vi "PropertyAdd.vi"(0 "Data":T1, 5 "error in":errorcluster) -> (14 "Data 2":T1, 19 "error out":errorcluster)   [LabVIEW 2017]
doc: "<B>This VI is used for adding a new property to the Caps file.</B>"
uses:
  Ctrl/Type Tab.ctl
  Ctrl/compond commands.ctl
  Ctrl/User Input Cluster.ctl
  Ctrl/Property.ctl
  Ctrl/PhysicalChannel.ctl
  Ctrl/Bitfield.ctl
  Ctrl/Register.ctl
  Ctrl/ScaleType.ctl
  Ctrl/Scale.ctl
  Ctrl/EnumValue.ctl
  Ctrl/Enum.ctl
  Ctrl/Caps.ctl
  Ctrl/Data.ctl
panel:
  in  "Write a Range?":bool
  out "Lable":string
  in  "Write a Register?":bool
  in  "Scale method":u16(ring) items=["TableStrict", "TableStrict12Elements", "PolynomialBoundaryConditions", "PolynomialThermocouple", "Times2Plus2", "LinearDivideBy8", "TableInterpolate", "TableRound", "NoScale"]
  in  "Min":dbl
  in  "Max":dbl
  out "Data Range":T11
  in  "Min(Double)":dbl
  in  "Max(Double)":dbl
  in  "Max(U64)":u64
  in  "Min(U64)":u64
  in  "Min(I64)":i64
  in  "Max(I64)":i64
  in  "Max(U32)":u32
  in  "Min(U32)":u32
  in  "Min(I32)":i32
  in  "Max(I32)":i32
  in  "OK Button":bool
  in  "Documentation":string
  in  "String":string
  in  "U8":u8 format="%.0x"
  in  "I8":i8
  in  "U32":u32
  in  "I32":i32
  in  "U64":u64
  in  "I64":i64
  in  "Ring":u16(ring) items=["False", "True"]
  in  "DBL":dbl format="%#_16g"
  in  "Description":string
  in  "Access":u16(ring) items=["Read Only", "Write Only", "Read/Write"]
  in  "Bitfield":u16(ring) items=["DebugScratch8/ScratchI8", "DebugScratch8/Scratch8", "DebugScratch8/ScratchBool", "DebugScratch16/ScratchBool", "DebugScratch16/ScratchI8", "DebugScratch16/Scratch8", "DebugScratch16/ScratchI16", "DebugScratch16/Scratch16", "DebugScratch32/ScratchBool", "DebugScratch32/ScratchI8", "DebugScratch32/Scratch8", "DebugScratch32/ScratchI16", "DebugScratch32/Scratch16", "DebugScratch32/ScratchI32", "DebugScratch32/Scratch32", "DebugLeds/DebugLed3", "DebugLeds/DebugLed2", "DebugLeds/DebugLed1", "DebugLeds/DebugLed0", "DebugDipSwitch/DipSwitch8", "DebugDipSwitch/DipSwitch7", "DebugDipSwitch/DipSwitch6", "DebugDipSwitch/DipSwitch5", "DebugDipSwitch/DipSwitch4", "DebugDipSwitch/DipSwitch3", "DebugDipSwitch/DipSwitch2", "DebugDipSwitch/DipSwitch1", "DebugScratch64/ScratchBool", "DebugScratch64/ScratchI8", "DebugScratch64/Scratch8", "DebugScratch64/ScratchI16", "DebugScratch64/Scratch16", "DebugScratch64/ScratchI32", "DebugScratch64/Scratch32", "DebugScratch64/ScratchI64", "DebugScratch64/Scratch64", "FrontPanelLeds/LedRed0Enable", "FrontPanelLeds/LedRed1Enable", "FrontPanelLeds/LedRed2Enable", "FrontPanelLeds/LedGreen0Enable", "FrontPanelLeds/LedGreen1Enable", "FrontPanelLeds/LedGreen2Enable", "Revision/DateCode", "InterruptAck/EventIntAck0", "InterruptAck/EventIntAck1", "InterruptAck/EventIntAck2", "InterruptAck/EventIntAck3", "InterruptAck/ExternalIntAck0", "InterruptAck/ExternalIntAck1", "InterruptAck/ExternalIntAck2", "InterruptAck/ExternalIntAck3", "InterruptDisable/EventIntDisable0", "InterruptDisable/EventIntDisable1", "InterruptDisable/EventIntDisable2", "InterruptDisable/EventIntDisable3", "InterruptDisable/ExternalIntDisable0", "InterruptDisable/ExternalIntDisable1", "InterruptDisable/ExternalIntDisable2", "InterruptDisable/ExternalIntDisable3", "InterruptEnable/EventIntEnable0", "InterruptEnable/EventIntEnable1", "InterruptEnable/EventIntEnable2", "InterruptEnable/EventIntEnable3", "InterruptEnable/ExternalIntEnable0", "InterruptEnable/ExternalIntEnable1", "InterruptEnable/ExternalIntEnable2", "InterruptEnable/ExternalIntEnable3", "InterruptMask/EventIntMask0", "InterruptMask/EventIntMask1", "InterruptMask/EventIntMask2", "InterruptMask/EventIntMask3", "InterruptMask/ExternalIntMask0", "InterruptMask/ExternalIntMask1", "InterruptMask/ExternalIntMask2", "InterruptMask/ExternalIntMask3", "InterruptStatus/EventIntStatus0", "InterruptStatus/EventIntStatus1", "InterruptStatus/EventIntStatus2", "InterruptStatus/EventIntStatus3", "InterruptStatus/ExternalIntStatus0", "InterruptStatus/ExternalIntStatus1", "InterruptStatus/ExternalIntStatus2", "InterruptStatus/ExternalIntStatus3", "EventCounter3/DelayInMilliseconds", "EventCounter2/DelayInMilliseconds", "EventCounter1/DelayInMilliseconds", "EventCounter0/DelayInMilliseconds", "EventStartRegister/EventStart0", "EventStartRegister/EventStart1", "EventStartRegister/EventStart2", "EventStartRegister/EventStart3"]
  in  "DataType":T12(ring)
  in  "Name":string
  # "Value"
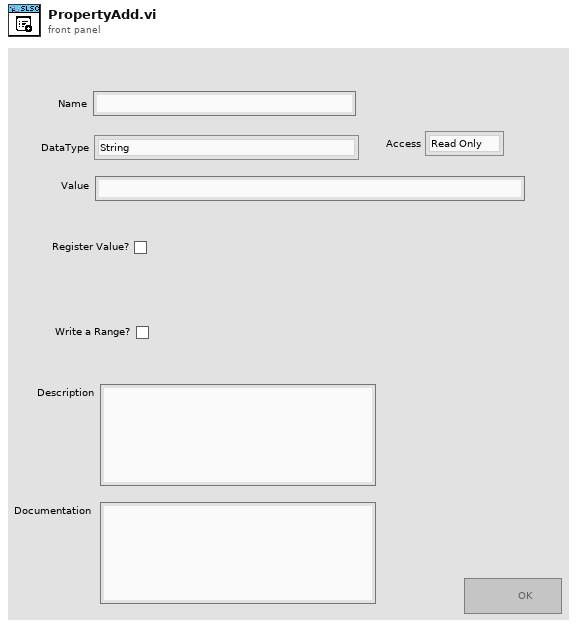
[diagram p1: front panel]
types:
  T1 = typedef "Data.ctl" = cluster{"Ref Cluster":cluster{"String":refnum<vi>, "U8":refnum<vi>, "I8":refnum<vi>, "U32":refnum<vi>, "I32":refnum<vi>, "U64":refnum<vi>, "I64":refnum<vi>, "Ring":refnum<vi>, "DBL":refnum<vi>, "Add":refnum<vi>, "Remove":refnum<vi>, "Property tree":refnum<vi>}, "JSON Text":string, "Original JSON Text":string, "Caps":T2, "SLSC Output Tree":cluster{"Left Cell String":string, "Child Text":string[], "Child Tag":string, "Item Indent":i32, "Child Only?":bool, "Glyph Index":i32, "offline value":variant}[], "Ref Index and Control Type":cluster{"index":i32, "Datatype":string}, "Selected Type and name":cluster{"Selected Type":enum16{"Property", "Physical Channel"}, "Selected Property Name":string}, "Update whole Tree?":bool}
  T2 = typedef "Caps.ctl" = cluster{"properties":T3[], "physical channels":T4[], "registers":T5[], "scales":T7[], "enums":T9[], "productName":string}
  T3 = typedef "Property.ctl" = cluster{"name":string, "bitfield":string, "value":variant, "dataType":string, "min":variant, "max":variant, "scale":string, "access":string}
  T4 = typedef "PhysicalChannel.ctl" = cluster{"name":string, "properties":T3[]}
  T5 = typedef "Register.ctl" = cluster{"name":string, "address":i32, "size":i32, "bitfields":T6[], "initialValue":variant, "connectedProperties":string[]}
  T6 = typedef "Bitfield.ctl" = cluster{"name":string, "offset":i32, "size":i32, "signed":bool}
  T7 = typedef "Scale.ctl" = cluster{"name":string, "type":T8, "params":variant}
  T8 = typedef "ScaleType.ctl" = enum16{"NoScale", "Table", "Polynomial", "Linear"}
  T9 = typedef "Enum.ctl" = cluster{"name":string, "values":T10[]}
  T10 = typedef "EnumValue.ctl" = cluster{"name":string, "value":i32}
  T11 = typedef "Type Tab.ctl" = enum32{"String", "Double", "U64", "I64", "U32", "I32", "Bool"}
  T12 = enum16{"String", "Double", "U64", "I64", "U32", "I32", "Bool"}
  T13 = typedef "User Input Cluster.ctl" = cluster{"Name":string, "DataType":enum16{"String", "Double", "U64", "I64", "U32", "I32", "Bool"}, "Bitfield":u16, "Access":u16, "Description":string, "Documentation":string, "Min_Max_Cluster":cluster{"Min(Double)":dbl, "Max(Double)":dbl, "Min(U64)":u64, "Max(U64)":u64, "Min(I64)":i64, "Max(I64)":i64, "Min(U32)":u32, "Max(U32)":u32, "Min(I32)":i32, "Max(I32)":i32}, "Value Cluster":cluster{"DBL":dbl, "Ring":u16, "I64":i64, "U64":u64, "I32":i32, "U32":u32, "I8":i8, "U8":u8, "String":string}, "Scale method list":u16}
  T14 = cluster{"DBL":dbl, "Ring":u16, "I64":i64, "U64":u64, "I32":i32, "U32":u32, "I8":i8, "U8":u8, "String":string}
  T15 = cluster{"Min(Double)":dbl, "Max(Double)":dbl, "Min(U64)":u64, "Max(U64)":u64, "Min(I64)":i64, "Max(I64)":i64, "Min(U32)":u32, "Max(U32)":u32, "Min(I32)":i32, "Max(I32)":i32}
  T16 = enum8{"Enabled", "Disabled", "Disabled and Grayed Out"}
  T17 = typedef "compond commands.ctl" = enum16{"Get Property Array", "Get Physical Channel Property Array", "Get the Selected Position", "Get Property and Physical Channel Name", "Get Type and Value", "Make and Set a new Property", "Modify the Value", "Delete a Property"}
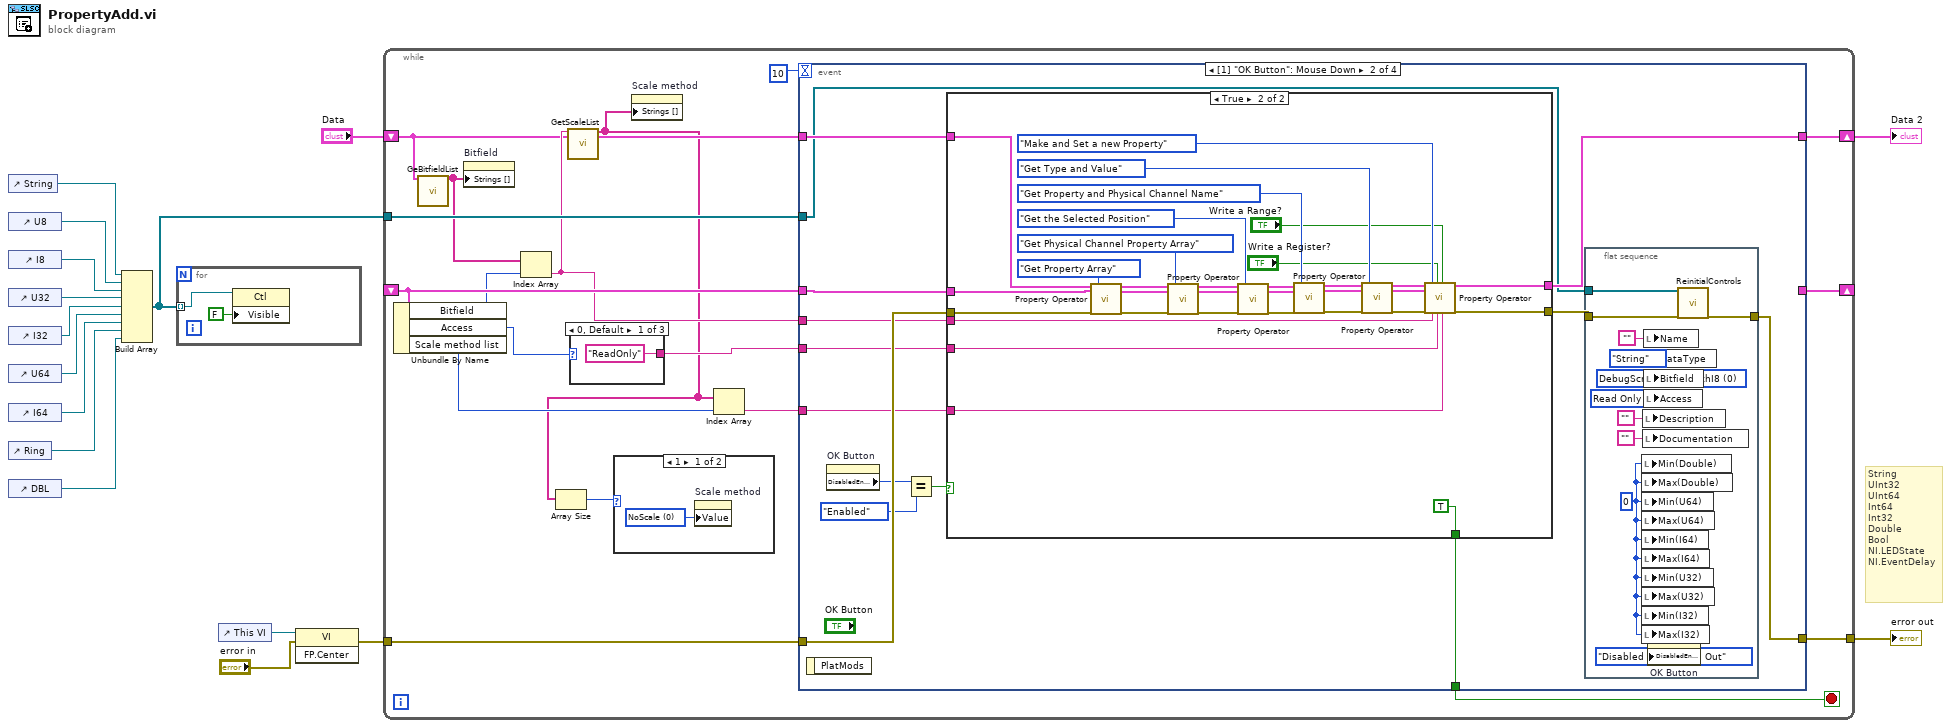
[diagram p0: block diagram]
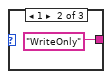
[diagram p3: hidden frame]
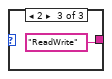
[diagram p4: hidden frame]
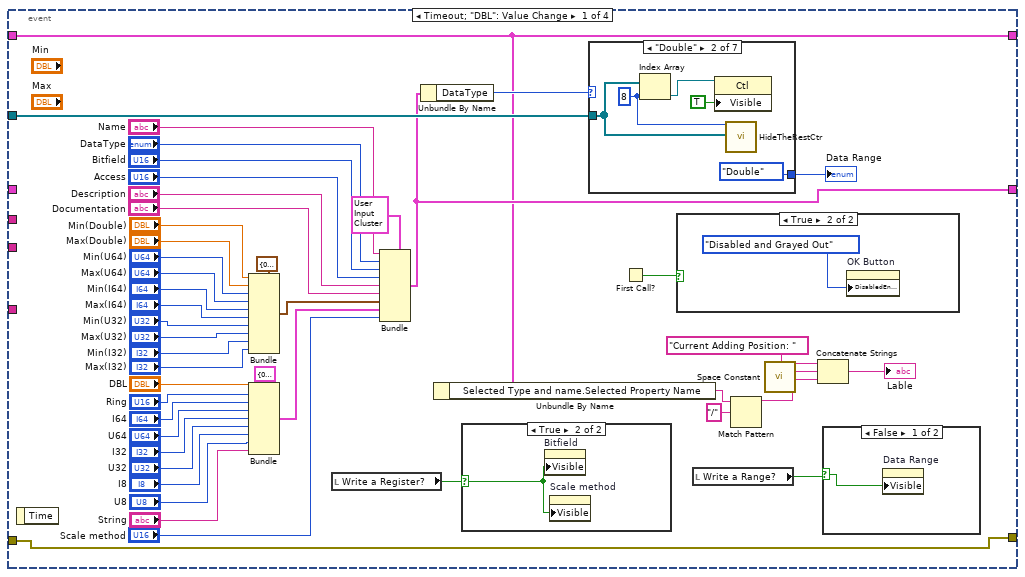
[diagram p5: hidden frame]
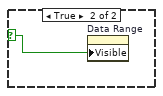
[diagram p6: hidden frame]
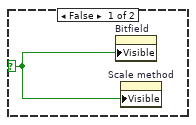
[diagram p7: hidden frame]
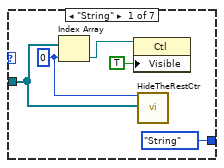
[diagram p9: hidden frame]
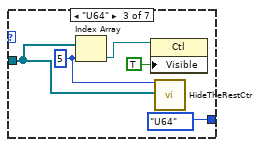
[diagram p10: hidden frame]
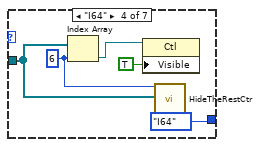
[diagram p11: hidden frame]
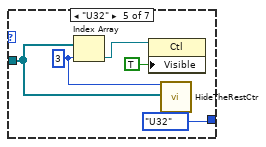
[diagram p12: hidden frame]
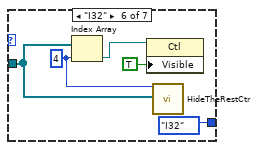
[diagram p13: hidden frame]
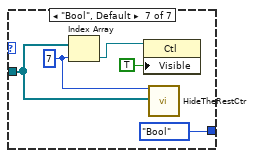
[diagram p14: hidden frame]
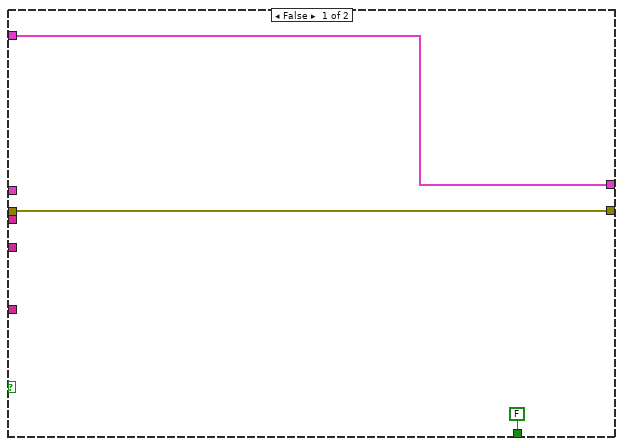
[diagram p15: hidden frame]
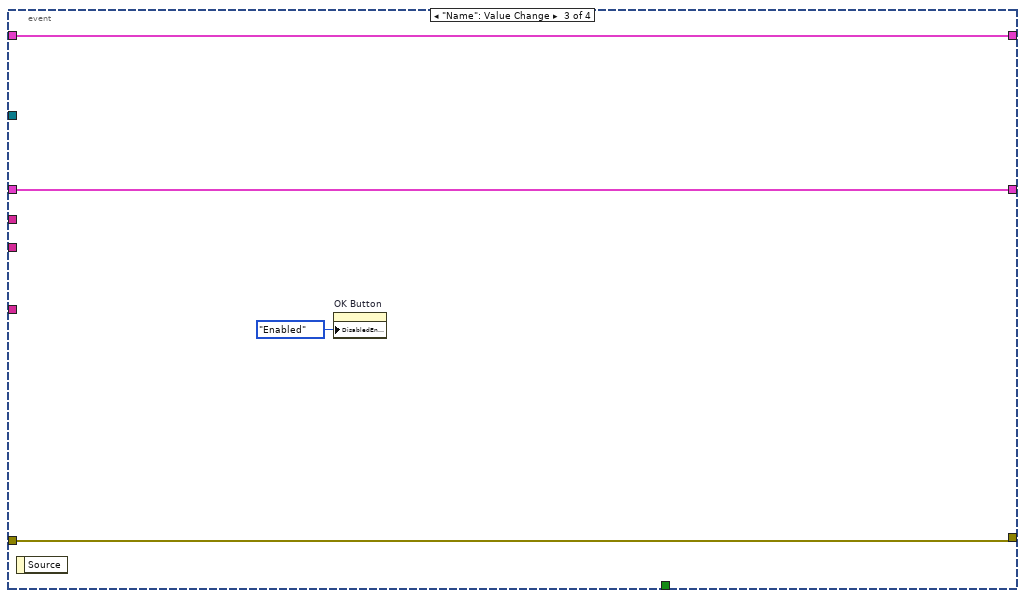
[diagram p16: hidden frame]
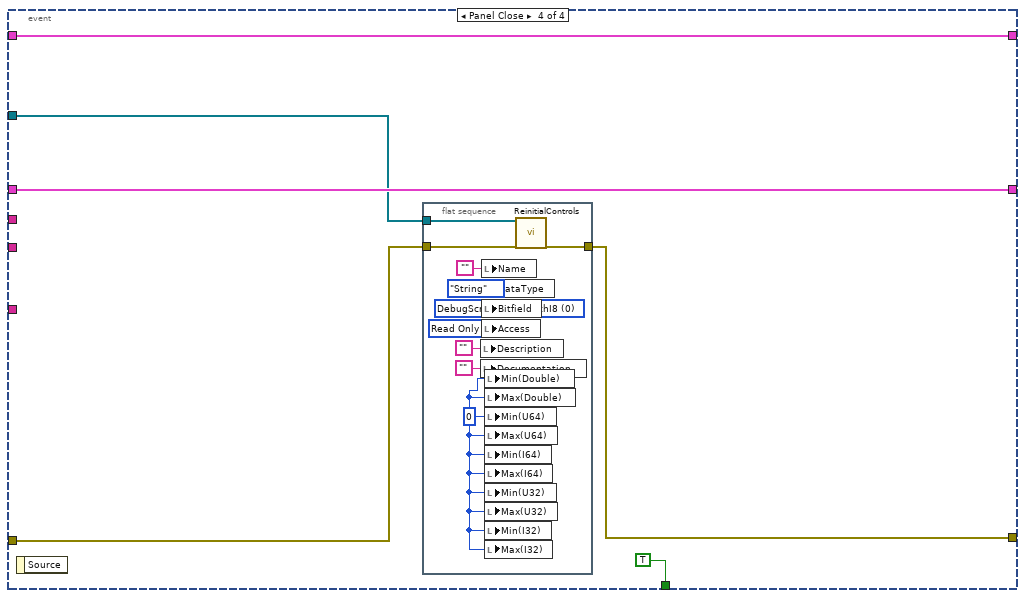
[diagram p17: hidden frame]
diagram:
  # "String\nUInt32\nUInt64\nInt64\nInt32\nDouble\nBool\nNI.LEDState\nNI.EventDelay"
  n1 = control-ref of="String"() -> (w16:refnum<vi>)
  n2 = control-ref of="U8"() -> (w15:refnum<vi>)
  n3 = control-ref of="I8"() -> (w14:refnum<vi>)
  n4 = control-ref of="U32"() -> (w13:refnum<vi>)
  n5 = control-ref of="I32"() -> (w12:refnum<vi>)
  n6 = control-ref of="U64"() -> (w11:refnum<vi>)
  n7 = control-ref of="I64"() -> (w10:refnum<vi>)
  n8 = control-ref of="Ring"() -> (w9:refnum<vi>)
  n9 = control-ref of="DBL"() -> (w8:refnum<vi>)
  n10 = Build Array(w16, w15, w14, w13, w12, w11, w10, w9, w8) -> (w1:refnum<vi>[])
  n11 = for {
    tunnel: w1 -> [w18] mode=indexing
    n12 = property class="Ctl"(reference=w18, "Visible"=FALSE) -> ()  [unwired: 1 in, 2 out]
  }
  n13 = control-ref of="This VI"() -> (w4:refnum<vi>)
  n14 = invoke class="VI" method="FP.Center"(reference=w4, error in="error in") -> (error out=w3:errorcluster)  [unwired: 1 in, 2 out]
  n15 = while {
    tunnel: w1 -> [w34]
    tunnel: w3 -> [w35]
    tunnel: [w36] -> w7
    shift-right: [w37] -> w5
    shift-left: "Data" -> [w25]
    shift-right: [w32] -> _
    shift-left: _ -> [w31]
    stop <- w19 stop-if-true
    n16 = Unbundle By Name(w31) -> ("Bitfield"=w30:u16, "Access"=w29:u16, "Scale method list"=w23:u16)
    n17 = call "GeBitfieldList.vi"("Data"=w25) -> ("Array"=w24:string[])  [unwired: 18 in]
    n18 = property on="Bitfield" class="Ring (strict)"("Strings []"=w24) -> ()  [unwired: 2 in, 2 out]
    n19 = Index Array(array=w24, index=w30) -> (element=w28:string)
    n20 = call "GetScaleList.vi"("Bitfield in"=w28, "Data in"=w25) -> ("output array"=w21:string[], "Data out"=w26:T1)  [unwired: 16 in]
    n21 = Array Size(array=w21) -> (size(s)=w20:i32)
    n22 = case shown="0, Default" w29 {
      tunnel: ["ReadOnly" "WriteOnly" "ReadWrite"] -> w27
      frame 0, Default {
      }
      frame 1 {
      }
      frame 2 {
      }
    }
    n23 = case shown="1" w20 {
      frame 1 {
        w38 = u16 0 items=["NoScale"] ("Scale method")
        n24 = property on="Scale method" class="Ring (strict)"("Value"=w38) -> ()  [unwired: 2 in, 2 out]
      }
      frame Default {
      }
    }
    n25 = property on="Scale method" class="Ring (strict)"("Strings []"=w21) -> ()  [unwired: 2 in, 2 out]
    n26 = Index Array(array=w21, index=w23) -> (element=w22:string)
    n27 = event shown="[1] \"OK Button\": Mouse Down" {
      selector: _ -> [_ _ _ _]
      dyn-events: _ -> [_ _ _ _]
      timeout: 10 -> [_ _ _ _]
      tunnel: w26 -> [w50 w140 w191 w197]
      tunnel: [w50 w139 w191 w197] -> w37
      tunnel: w35 -> [w51 w141 w188 w194]
      tunnel: [w51 w137 w188 w193] -> w36
      tunnel: w31 -> [_ w135 w190 w196]
      tunnel: w34 -> [w85 w136 _ w195]
      tunnel: [w56 _ w190 w196] -> w32
      tunnel: w28 -> [_ w134 _ _]
      tunnel: w27 -> [_ w133 _ _]
      tunnel: w22 -> [_ w132 _ _]
      tunnel: [_ w128 _ TRUE] -> w19
      event Timeout; "DBL": Value Change {
        n28 = event-data() -> ()  [unwired: 1 in, 1 out]
        n29 = Bundle(cluster=T15 {"Min(Double)"=0.0, "Max(Double)"=0.0, "Min(U64)"=0, "Max(U64)"=0, "Min(I64)"=0, "Max(I64)"=0, "Min(U32)"=0, "Max(U32)"=0, "Min(I32)"=0, "Max(I32)"=0} ("Min_Max_Cluster"), "Min(Double)"="Min(Double)", "Max(Double)"="Max(Double)", "Min(U64)"="Min(U64)", "Max(U64)"="Max(U64)", "Min(I64)"="Min(I64)", "Max(I64)"="Max(I64)", "Min(U32)"="Min(U32)", "Max(U32)"="Max(U32)", "Min(I32)"="Min(I32)", "Max(I32)"="Max(I32)") -> (w60:T15)
        n30 = Bundle(cluster=T14 {"DBL"=0.0, "Ring"=0, "I64"=0, "U64"=0, "I32"=0, "U32"=0, "I8"=0, "U8"=0, "String"=""} ("Value Cluster"), "DBL"="DBL", "Ring"="Ring", "I64"="I64", "U64"="U64", "I32"="I32", "U32"="U32", "I8"="I8", "U8"="U8", "String"="String") -> (w59:T14)
        n31 = local read "Write a Register?"() -> (w49:bool)
        n32 = Bundle(cluster=T13 {"Name"="", "DataType"=enum."String", "Bitfield"=0, "Access"=0, "Description"="", "Documentation"="", "Min_Max_Cluster"={"Min(Double)"=0.0, "Max(Double)"=0.0, "Min(U64)"=0, "Max(U64)"=0, "Min(I64)"=0, "Max(I64)"=0, "Min(U32)"=0, "Max(U32)"=0, "Min(I32)"=0, "Max(I32)"=0}, "Value Cluster"={"DBL"=0.0, "Ring"=0, "I64"=0, "U64"=0, "I32"=0, "U32"=0, "I8"=0, "U8"=0, "String"=""}, "Scale method list"=0}, "Name"="Name", "DataType"="DataType", "Bitfield"="Bitfield", "Access"="Access", "Description"="Description", "Documentation"="Documentation", "Min_Max_Cluster"=w60, "Value Cluster"=w59, "Scale method list"="Scale method") -> (w56:T13)
        n33 = Unbundle By Name(w56) -> ("DataType"=w86:T12)
        n34 = Unbundle By Name(w50) -> ("Selected Type and name.Selected Property Name"=w45:string)
        n35 = case shown="True" w49 {
          selector: w49 -> [w90 w91]
          frame False {
            n36 = property on="Bitfield" class="Ring (strict)"("Visible"=w90) -> ()  [unwired: 2 in, 2 out]
            n37 = property on="Scale method" class="Ring (strict)"("Visible"=w90) -> ()  [unwired: 2 in, 2 out]
          }
          frame True {
            n38 = property on="Bitfield" class="Ring (strict)"("Visible"=w91) -> ()  [unwired: 2 in, 2 out]
            n39 = property on="Scale method" class="Ring (strict)"("Visible"=w91) -> ()  [unwired: 2 in, 2 out]
          }
        }
        n40 = case shown="\"Double\"" w86 {
          tunnel: w85 -> [w94 w100 w104 w109 w114 w119 w124]
          tunnel: [Type_Tab."String" ("Tab Control") Type_Tab."Double" ("Tab Control") Type_Tab."U64" ("Tab Control") Type_Tab."I64" ("Tab Control") Type_Tab."U32" ("Tab Control") Type_Tab."I32" ("Tab Control") Type_Tab."Bool" ("Tab Control")] -> w87
          frame "String" {
            w95 = 0 ("index")
            n41 = Index Array(array=w94, index=w95) -> (element=w97:refnum<vi>)
            n42 = property class="Ctl"(reference=w97, "Visible"=TRUE) -> ()  [unwired: 1 in, 2 out]
            n43 = call "HideTheRestCtr.vi"("index"=w95, "Array"=w94) -> ()  [unwired: 18 in]
          }
          frame "Double" {
            w99 = 8 ("index")
            n44 = Index Array(array=w100, index=w99) -> (element=w102:refnum<vi>)
            n45 = property class="Ctl"(reference=w102, "Visible"=TRUE) -> ()  [unwired: 1 in, 2 out]
            n46 = call "HideTheRestCtr.vi"("index"=w99, "Array"=w100) -> ()  [unwired: 18 in]
          }
          frame "U64" {
            w105 = 5 ("index")
            n47 = Index Array(array=w104, index=w105) -> (element=w107:refnum<vi>)
            n48 = property class="Ctl"(reference=w107, "Visible"=TRUE) -> ()  [unwired: 1 in, 2 out]
            n49 = call "HideTheRestCtr.vi"("index"=w105, "Array"=w104) -> ()  [unwired: 18 in]
          }
          frame "I64" {
            w110 = 6 ("index")
            n50 = Index Array(array=w109, index=w110) -> (element=w112:refnum<vi>)
            n51 = property class="Ctl"(reference=w112, "Visible"=TRUE) -> ()  [unwired: 1 in, 2 out]
            n52 = call "HideTheRestCtr.vi"("index"=w110, "Array"=w109) -> ()  [unwired: 18 in]
          }
          frame "U32" {
            w115 = 3 ("index")
            n53 = Index Array(array=w114, index=w115) -> (element=w117:refnum<vi>)
            n54 = property class="Ctl"(reference=w117, "Visible"=TRUE) -> ()  [unwired: 1 in, 2 out]
            n55 = call "HideTheRestCtr.vi"("index"=w115, "Array"=w114) -> ()  [unwired: 18 in]
          }
          frame "I32" {
            w120 = 4 ("index")
            n56 = Index Array(array=w119, index=w120) -> (element=w122:refnum<vi>)
            n57 = property class="Ctl"(reference=w122, "Visible"=TRUE) -> ()  [unwired: 1 in, 2 out]
            n58 = call "HideTheRestCtr.vi"("index"=w120, "Array"=w119) -> ()  [unwired: 18 in]
          }
          frame "Bool", Default {
            w125 = 7 ("index")
            n59 = Index Array(array=w124, index=w125) -> (element=w127:refnum<vi>)
            n60 = property class="Ctl"(reference=w127, "Visible"=TRUE) -> ()  [unwired: 1 in, 2 out]
            n61 = call "HideTheRestCtr.vi"("index"=w125, "Array"=w124) -> ()  [unwired: 18 in]
          }
        }
        "Data Range" <- w87
        n62 = First Call?() -> (First Call?: T/F=w84:bool)
        n63 = case shown="True" w84 {
          frame False {
          }
          frame True {
            n64 = property on="OK Button" class="Bool (strict)"("DisabledEnum"=T16."Disabled and Grayed Out" ("Disabled")) -> ()  [unwired: 2 in, 2 out]
          }
        }
        n65 = local read "Write a Range?"() -> (w42:bool)
        n66 = Match Pattern(string=w45, regular expression="/") -> (before substring=w43:string)  [unwired: 1 in, 3 out]
        n67 = call <vilib>:"Space Constant.vi"() -> ("String"=w46:string)
        n68 = Concatenate Strings("Current Adding Position: " ("string"), w46, w43) -> (→"Lable":string)
        n69 = case shown="False" w42 {
          selector: w42 -> [w88 w89]
          frame False {
            n70 = property on="Data Range" class="TabCtl (strict)"("Visible"=w88) -> ()  [unwired: 2 in, 2 out]
          }
          frame True {
            n71 = property on="Data Range" class="TabCtl (strict)"("Visible"=w89) -> ()  [unwired: 2 in, 2 out]
          }
        }
      }
      event "OK Button": Mouse Down {
        n72 = event-data() -> ()  [unwired: 1 in, 1 out]
        n73 = property on="OK Button" class="Bool (strict)"() -> ("DisabledEnum"=w130:T16)  [unwired: 2 in, 2 out]
        n74 = Equal?(x=w130, y=T16."Enabled") -> (x = y?=w131:bool)
        n75 = case shown="True" w131 {
          tunnel: w141 -> [w143 w170]
          tunnel: w140 -> [w144 w165]
          tunnel: [w144 w149] -> w139
          tunnel: [w143 w148] -> w138
          tunnel: w135 -> [_ w164]
          tunnel: w134 -> [_ w147]
          tunnel: w133 -> [_ w146]
          tunnel: w132 -> [_ w145]
          tunnel: [FALSE TRUE] -> w128
          frame False {
          }
          frame True {
            n76 = call "Property Operator.vi"("Data"=w165, "User Input"=w164, "error in"=w170, "Command"=compond_commands."Get Property Array") -> ("Data 2"=w176:T1, "User Input 2"=w163:T13, "error out"=w175:errorcluster)  [unwired: 12 in, 1 out]
            n77 = call "Property Operator.vi"("Data"=w176, "User Input"=w163, "error in"=w175, "Command"=compond_commands."Get Physical Channel Property Array") -> ("Data 2"=w174:T1, "User Input 2"=w162:T13, "error out"=w173:errorcluster)  [unwired: 12 in, 1 out]
            n78 = call "Property Operator.vi"("Data"=w174, "User Input"=w162, "error in"=w173, "Command"=compond_commands."Get the Selected Position") -> ("Data 2"=w172:T1, "User Input 2"=w161:T13, "error out"=w171:errorcluster)  [unwired: 12 in, 1 out]
            n79 = call "Property Operator.vi"("Data"=w172, "User Input"=w161, "error in"=w171, "Command"=compond_commands."Get Property and Physical Channel Name") -> ("Data 2"=w159:T1, "User Input 2"=w158:T13, "error out"=w157:errorcluster)  [unwired: 12 in, 1 out]
            n80 = call "Property Operator.vi"("Data"=w159, "User Input"=w158, "error in"=w157, "Command"=compond_commands."Get Type and Value") -> ("Data 2"=w155:T1, "User Input 2"=w154:T13, "error out"=w153:errorcluster)  [unwired: 12 in, 1 out]
            n81 = call "Property Operator.vi"("Data"=w155, "User Input"=w154, "error in"=w153, "Command"=compond_commands."Make and Set a new Property", "Bitfield"=w147, "Write a Register?"="Write a Register?", "Access"=w146, "Write a Range?"="Write a Range?", "Scale Method"=w145) -> ("Data 2"=w149:T1, "error out"=w148:errorcluster)  [unwired: 7 in, 2 out]
          }
        }
        n82 = flat-sequence {
          tunnel: w138 -> [w187]
          tunnel: [w186] -> w137
          tunnel: w136 -> [w185]
          frame #0 {
            w178 = u64 0 ("Min(U64)")
            w181 = u16 0 items=["Read Only", "Write Only", "Read/Write"] ("Access")
            w182 = u16 0 items=["DebugScratch8/ScratchI8", "DebugScratch8/Scratch8", "DebugScratch8/ScratchBool", "DebugScratch16/ScratchBool", "DebugScratch16/ScratchI8", "DebugScratch16/Scratch8", "DebugScratch16/ScratchI16", "DebugScratch16/Scratch16", "DebugScratch32/ScratchBool", "DebugScratch32/ScratchI8", "DebugScratch32/Scratch8", "DebugScratch32/ScratchI16", "DebugScratch32/Scratch16", "DebugScratch32/ScratchI32", "DebugScratch32/Scratch32", "DebugLeds/DebugLed3", "DebugLeds/DebugLed2", "DebugLeds/DebugLed1", "DebugLeds/DebugLed0", "DebugDipSwitch/DipSwitch8", "DebugDipSwitch/DipSwitch7", "DebugDipSwitch/DipSwitch6", "DebugDipSwitch/DipSwitch5", "DebugDipSwitch/DipSwitch4", "DebugDipSwitch/DipSwitch3", "DebugDipSwitch/DipSwitch2", "DebugDipSwitch/DipSwitch1", "DebugScratch64/ScratchBool", "DebugScratch64/ScratchI8", "DebugScratch64/Scratch8", "DebugScratch64/ScratchI16", "DebugScratch64/Scratch16", "DebugScratch64/ScratchI32", "DebugScratch64/Scratch32", "DebugScratch64/ScratchI64", "DebugScratch64/Scratch64", "FrontPanelLeds/LedRed0Enable", "FrontPanelLeds/LedRed1Enable", "FrontPanelLeds/LedRed2Enable", "FrontPanelLeds/LedGreen0Enable", "FrontPanelLeds/LedGreen1Enable", "FrontPanelLeds/LedGreen2Enable", "Revision/DateCode", "InterruptAck/EventIntAck0", "InterruptAck/EventIntAck1", "InterruptAck/EventIntAck2", "InterruptAck/EventIntAck3", "InterruptAck/ExternalIntAck0", "InterruptAck/ExternalIntAck1", "InterruptAck/ExternalIntAck2", "InterruptAck/ExternalIntAck3", "InterruptDisable/EventIntDisable0", "InterruptDisable/EventIntDisable1", "InterruptDisable/EventIntDisable2", "InterruptDisable/EventIntDisable3", "InterruptDisable/ExternalIntDisable0", "InterruptDisable/ExternalIntDisable1", "InterruptDisable/ExternalIntDisable2", "InterruptDisable/ExternalIntDisable3", "InterruptEnable/EventIntEnable0", "InterruptEnable/EventIntEnable1", "InterruptEnable/EventIntEnable2", "InterruptEnable/EventIntEnable3", "InterruptEnable/ExternalIntEnable0", "InterruptEnable/ExternalIntEnable1", "InterruptEnable/ExternalIntEnable2", "InterruptEnable/ExternalIntEnable3", "InterruptMask/EventIntMask0", "InterruptMask/EventIntMask1", "InterruptMask/EventIntMask2", "InterruptMask/EventIntMask3", "InterruptMask/ExternalIntMask0", "InterruptMask/ExternalIntMask1", "InterruptMask/ExternalIntMask2", "InterruptMask/ExternalIntMask3", "InterruptStatus/EventIntStatus0", "InterruptStatus/EventIntStatus1", "InterruptStatus/EventIntStatus2", "InterruptStatus/EventIntStatus3", "InterruptStatus/ExternalIntStatus0", "InterruptStatus/ExternalIntStatus1", "InterruptStatus/ExternalIntStatus2", "InterruptStatus/ExternalIntStatus3", "EventCounter3/DelayInMilliseconds", "EventCounter2/DelayInMilliseconds", "EventCounter1/DelayInMilliseconds", "EventCounter0/DelayInMilliseconds", "EventStartRegister/EventStart0", "EventStartRegister/EventStart1", "EventStartRegister/EventStart2", "EventStartRegister/EventStart3"] ("Bitfield")
            n83 = local write "Min(Double)"(w178) -> ()
            n84 = local write "Max(Double)"(w178) -> ()
            n85 = local write "Min(U64)"(w178) -> ()
            n86 = local write "Max(U64)"(w178) -> ()
            n87 = local write "Min(I64)"(w178) -> ()
            n88 = local write "Max(I64)"(w178) -> ()
            n89 = local write "Min(U32)"(w178) -> ()
            n90 = local write "Max(U32)"(w178) -> ()
            n91 = local write "Min(I32)"(w178) -> ()
            n92 = local write "Max(I32)"(w178) -> ()
            n93 = local write "Description"("" ("Description")) -> ()
            n94 = local write "Documentation"("" ("Documentation")) -> ()
            n95 = local write "Name"("" ("Name")) -> ()
            n96 = local write "DataType"(T12."String" ("DataType")) -> ()
            n97 = local write "Bitfield"(w182) -> ()
            n98 = local write "Access"(w181) -> ()
            n99 = property on="OK Button" class="Bool (strict)"("DisabledEnum"=T16."Disabled and Grayed Out" ("Disabled")) -> ()  [unwired: 2 in, 2 out]
            n100 = call "ReinitialControls.vi"("Array"=w185, "error in (no error)"=w187) -> ("error out"=w186:errorcluster)  [unwired: 17 in]
          }
        }
      }
      event "Name": Value Change {
        n101 = event-data() -> ()  [unwired: 1 in, 1 out]
        n102 = property on="OK Button" class="Bool (strict)"("DisabledEnum"=T16."Enabled" ("Disabled")) -> ()  [unwired: 2 in, 2 out]
      }
      event Panel Close {
        n103 = event-data() -> ()  [unwired: 1 in, 1 out]
        n104 = flat-sequence {
          tunnel: w194 -> [w207]
          tunnel: [w206] -> w193
          tunnel: w195 -> [w205]
          frame #0 {
            w198 = u64 0 ("Min(U64)")
            w201 = u16 0 items=["Read Only", "Write Only", "Read/Write"] ("Access")
            w202 = u16 0 items=["DebugScratch8/ScratchI8", "DebugScratch8/Scratch8", "DebugScratch8/ScratchBool", "DebugScratch16/ScratchBool", "DebugScratch16/ScratchI8", "DebugScratch16/Scratch8", "DebugScratch16/ScratchI16", "DebugScratch16/Scratch16", "DebugScratch32/ScratchBool", "DebugScratch32/ScratchI8", "DebugScratch32/Scratch8", "DebugScratch32/ScratchI16", "DebugScratch32/Scratch16", "DebugScratch32/ScratchI32", "DebugScratch32/Scratch32", "DebugLeds/DebugLed3", "DebugLeds/DebugLed2", "DebugLeds/DebugLed1", "DebugLeds/DebugLed0", "DebugDipSwitch/DipSwitch8", "DebugDipSwitch/DipSwitch7", "DebugDipSwitch/DipSwitch6", "DebugDipSwitch/DipSwitch5", "DebugDipSwitch/DipSwitch4", "DebugDipSwitch/DipSwitch3", "DebugDipSwitch/DipSwitch2", "DebugDipSwitch/DipSwitch1", "DebugScratch64/ScratchBool", "DebugScratch64/ScratchI8", "DebugScratch64/Scratch8", "DebugScratch64/ScratchI16", "DebugScratch64/Scratch16", "DebugScratch64/ScratchI32", "DebugScratch64/Scratch32", "DebugScratch64/ScratchI64", "DebugScratch64/Scratch64", "FrontPanelLeds/LedRed0Enable", "FrontPanelLeds/LedRed1Enable", "FrontPanelLeds/LedRed2Enable", "FrontPanelLeds/LedGreen0Enable", "FrontPanelLeds/LedGreen1Enable", "FrontPanelLeds/LedGreen2Enable", "Revision/DateCode", "InterruptAck/EventIntAck0", "InterruptAck/EventIntAck1", "InterruptAck/EventIntAck2", "InterruptAck/EventIntAck3", "InterruptAck/ExternalIntAck0", "InterruptAck/ExternalIntAck1", "InterruptAck/ExternalIntAck2", "InterruptAck/ExternalIntAck3", "InterruptDisable/EventIntDisable0", "InterruptDisable/EventIntDisable1", "InterruptDisable/EventIntDisable2", "InterruptDisable/EventIntDisable3", "InterruptDisable/ExternalIntDisable0", "InterruptDisable/ExternalIntDisable1", "InterruptDisable/ExternalIntDisable2", "InterruptDisable/ExternalIntDisable3", "InterruptEnable/EventIntEnable0", "InterruptEnable/EventIntEnable1", "InterruptEnable/EventIntEnable2", "InterruptEnable/EventIntEnable3", "InterruptEnable/ExternalIntEnable0", "InterruptEnable/ExternalIntEnable1", "InterruptEnable/ExternalIntEnable2", "InterruptEnable/ExternalIntEnable3", "InterruptMask/EventIntMask0", "InterruptMask/EventIntMask1", "InterruptMask/EventIntMask2", "InterruptMask/EventIntMask3", "InterruptMask/ExternalIntMask0", "InterruptMask/ExternalIntMask1", "InterruptMask/ExternalIntMask2", "InterruptMask/ExternalIntMask3", "InterruptStatus/EventIntStatus0", "InterruptStatus/EventIntStatus1", "InterruptStatus/EventIntStatus2", "InterruptStatus/EventIntStatus3", "InterruptStatus/ExternalIntStatus0", "InterruptStatus/ExternalIntStatus1", "InterruptStatus/ExternalIntStatus2", "InterruptStatus/ExternalIntStatus3", "EventCounter3/DelayInMilliseconds", "EventCounter2/DelayInMilliseconds", "EventCounter1/DelayInMilliseconds", "EventCounter0/DelayInMilliseconds", "EventStartRegister/EventStart0", "EventStartRegister/EventStart1", "EventStartRegister/EventStart2", "EventStartRegister/EventStart3"] ("Bitfield")
            n105 = local write "Description"("" ("Description")) -> ()
            n106 = local write "Documentation"("" ("Documentation")) -> ()
            n107 = local write "Name"("" ("Name")) -> ()
            n108 = local write "DataType"(T12."String" ("DataType")) -> ()
            n109 = local write "Bitfield"(w202) -> ()
            n110 = local write "Access"(w201) -> ()
            n111 = local write "Min(Double)"(w198) -> ()
            n112 = local write "Max(Double)"(w198) -> ()
            n113 = local write "Min(U64)"(w198) -> ()
            n114 = local write "Max(U64)"(w198) -> ()
            n115 = local write "Min(I64)"(w198) -> ()
            n116 = local write "Max(I64)"(w198) -> ()
            n117 = local write "Min(U32)"(w198) -> ()
            n118 = local write "Max(U32)"(w198) -> ()
            n119 = local write "Min(I32)"(w198) -> ()
            n120 = local write "Max(I32)"(w198) -> ()
            n121 = call "ReinitialControls.vi"("Array"=w205, "error in (no error)"=w207) -> ("error out"=w206:errorcluster)  [unwired: 17 in]
          }
        }
      }
    }
  }
  "error out" <- w7
  "Data 2" <- w5
